vi "Core Actor - CLOSE  - ALL Control References.vi"(8 "error in (no error)":errorcluster, 11 "Parent_Class in":refnum<class "Message_Distributor_Class.lvclass">) -> (0 "error out":errorcluster, 3 "Parent_Class out":refnum<class "Message_Distributor_Class.lvclass">)   [LabVIEW 2023, in "Actor_Message_Distributor.lvlib" / "Message_Distributor_Class.lvclass"]
uses:
  Message_Distributor_Class.lvclass
  Message_Distributor_Class.lvclass/Message_Distributor_Class.ctl
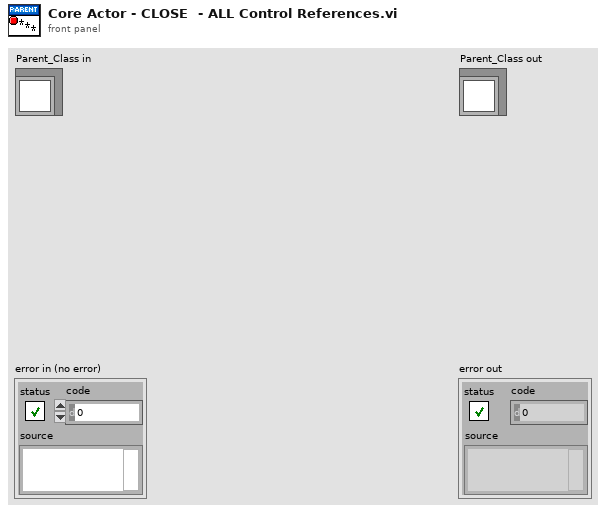
[diagram p1: front panel]
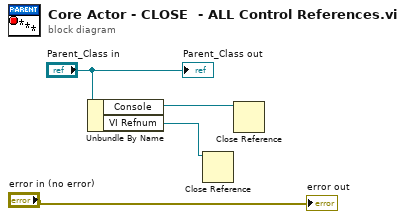
[diagram p0: block diagram]
diagram:
  n1 = Unbundle By Name("Parent_Class in") -> ("Console"=w3:refnum<vi>, "VI Refnum"=w2:refnum<vi>)
  n2 = Close Reference(reference=w2) -> ()  [unwired: 1 in, 1 out]
  n3 = Close Reference(reference=w3) -> ()  [unwired: 1 in, 1 out]
  "error out" <- "error in (no error)"
  "Parent_Class out" <- "Parent_Class in"
